vi "GetMyClassAttribute.vi"(5 "error in (no error)":errorcluster) -> (15 "MyClassAttribute":dbl, 19 "error out":errorcluster)   [LabVIEW 2017, in "MyStaticClass.lvclass"]
uses:
  MyStaticClass.lvclass
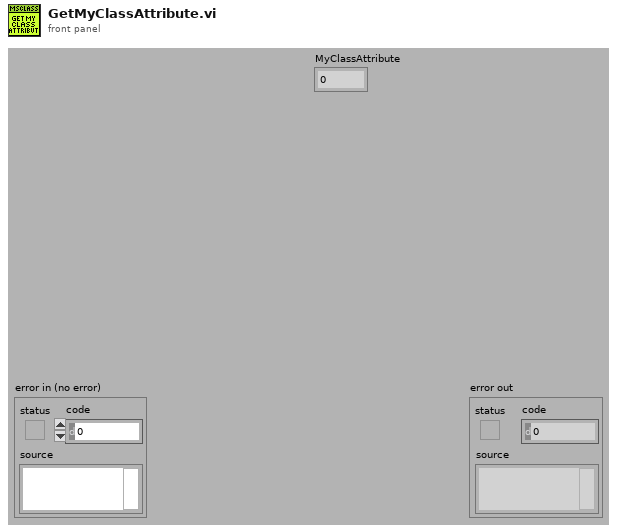
[diagram p1: front panel]
types:
  T1 = typedef "MyStaticClass.lvclass/ClassAttributes.ctl" = cluster{"MyClassAttribute":dbl}
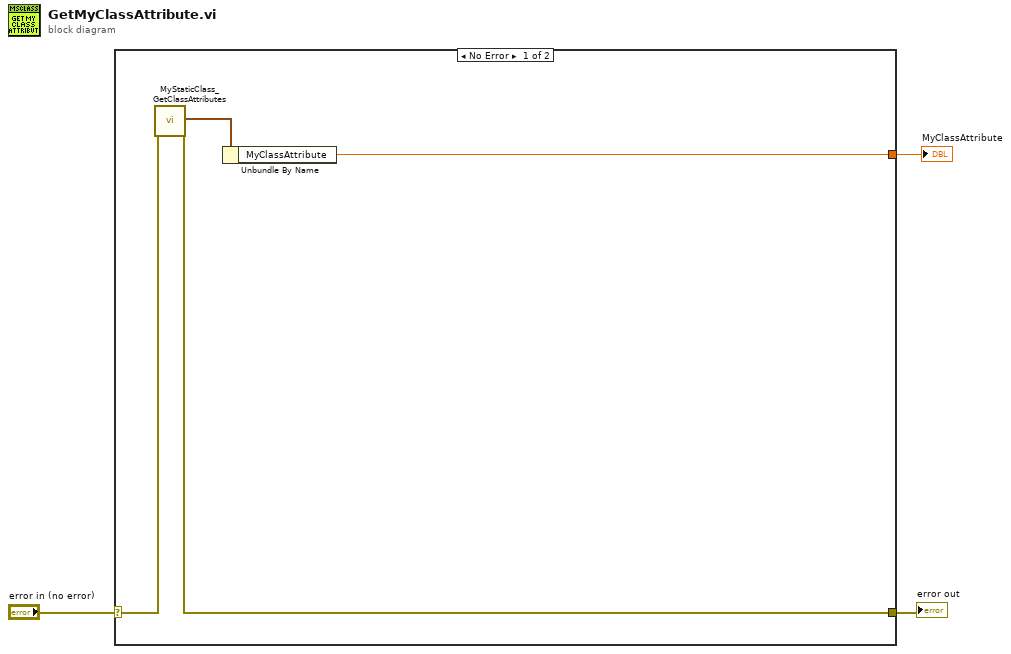
[diagram p0: block diagram]
diagram:
  n1 = case shown="No Error" "error in (no error)" {
    selector: "error in (no error)" -> [w7 w8]
    tunnel: [w6 w8] -> w2
    tunnel: [w4 _] -> w1
    frame No Error {
      n2 = call "MyStaticClass_GetClassAttributes.vi"("error in (no error)"=w7) -> ("class attributes"=w5:T1, "error out"=w6:errorcluster)  [unwired: 15 in, 2 out]
      n3 = Unbundle By Name(w5) -> ("MyClassAttribute"=w4:dbl)
    }
    frame Error {
    }
  }
  "error out" <- w2
  "MyClassAttribute" <- w1
